vi "lv dataset free.vi"(8 "error in":errorcluster, 11 "dataset handle":i32) -> (0 "error out":errorcluster)   [LabVIEW 2026]
uses:
  bin/nominalClient_64.dll
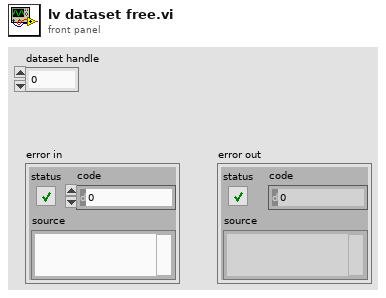
[diagram p1: front panel]
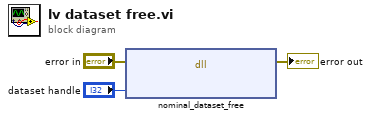
[diagram p0: block diagram]
diagram:
  n1 = dll-call lib="C:/sw/nominal-c/bin/nominalClient_64.dll" fn="nominal_dataset_free"(error in="error in", "dataset handle"="dataset handle") -> (error out=→"error out":errorcluster)  [unwired: 4 in, 1 out]
